vi "2020-IntakeMotor.vi"(8 "error in":errorcluster, 11 "Boolean":bool) -> (0 "error out":errorcluster)   [LabVIEW 2020]
uses:
  2020LabView/2020-Robot Global Data.vi
  <vilib>/Rock Robotics/WPI/ThirdParty/Phoenix-LabVIEW/Motor Controller/Controls/CTRE_Phoenix_MotorControl_ControlMode.ctl
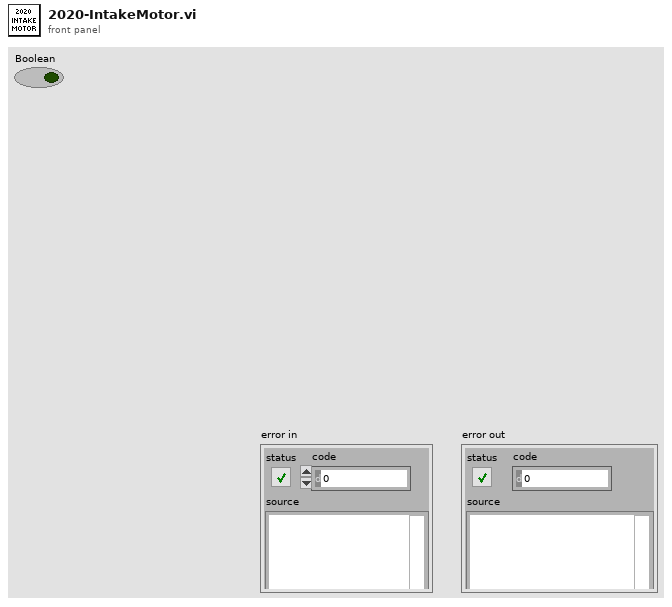
[diagram p1: front panel]
types:
  T1 = typedef "CTRE_Phoenix_MotorControl_ControlMode.ctl" = u16
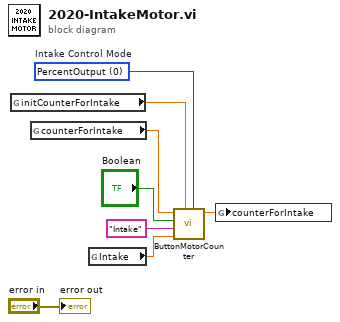
[diagram p0: block diagram]
diagram:
  w1 = T1 0 items=["PercentOutput"=0, "Position"=1, "Velocity"=2, "Current"=3, "Follower"=5, "MotionProfile"=6, "MotionMagic"=7, "MotionProfileArc"=10, "Disabled"=15]  # Intake Control Mode
  n1 = global read "2020-Robot Global Data.vi" "initCounterForIntake"() -> (w7:dbl)
  n2 = global read "2020-Robot Global Data.vi" "counterForIntake"() -> (w5:dbl)
  n3 = global read "2020-Robot Global Data.vi" "Intake"() -> (w6:dbl)
  n4 = call "ButtonMotorCounter.vi"("Motor Controller Control Mode"=w1, "counterStartValue"=w7, "Motor Set Point"=w6, "refnum name"="Intake", "Boolean"="Boolean", "counterForIntake in"=w5) -> ("counterForIntake out"=w4:dbl)  [unwired: 4 in, 1 out]
  n5 = global write "2020-Robot Global Data.vi" "counterForIntake"(w4) -> ()
  "error out" <- "error in"
